vi "Exporting VIs.vi"() -> ()   [LabVIEW 2019]
doc: "This example connects to a server VI that is exporting other VIs through VI Server. It shows how you might browse from one or more applications that may be exporting data from one or more data stations. \n\nThe example shows how to get references to exported VIs and call them with the Call By Reference function."
panel:
  in  "VIs to Export":string="VIs to Export"
  in  "Stop":bool
  out "Data":dbl[](graph)
  in  "Exported VI":i32(listbox)
  # "Overview: Illustrates how to configure and execute Exported VIs in VI Server.\nInstructions:\n1. Ensure Tools > Options > VI Server > Protocols > TCP/IP is enabled, and Port is set to '3363'.\n2. Run the VI. The server VI will open.\n3. Change the Exported VI option below to see the output of different VIs exported by the server displayed in the Data graph.\n4. Click Stop to stop this VI.\n5. Click Stop Server in the server VI to stop the server."
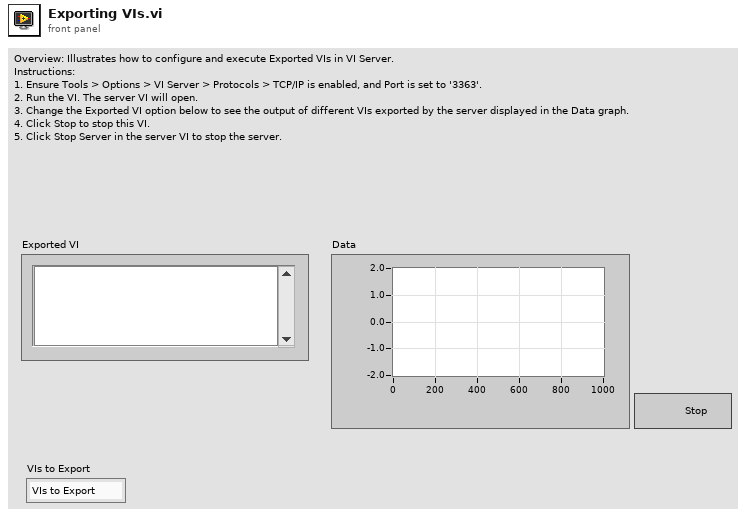
[diagram p1: front panel]
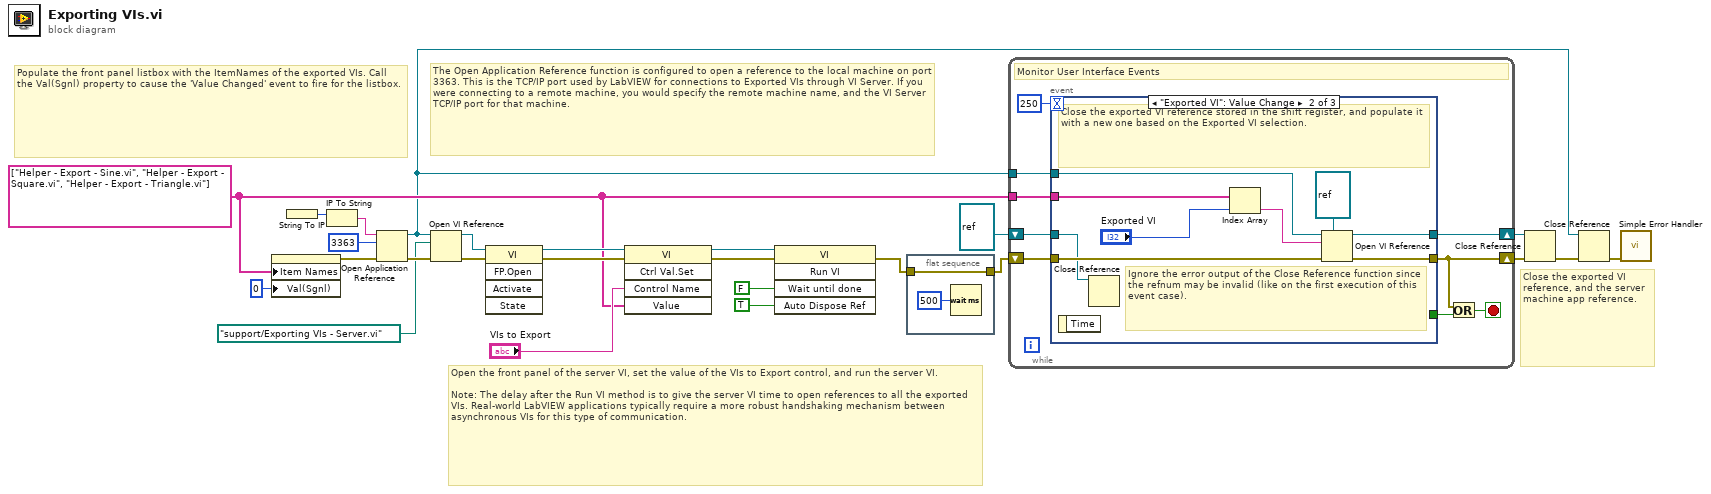
[diagram p0: block diagram]
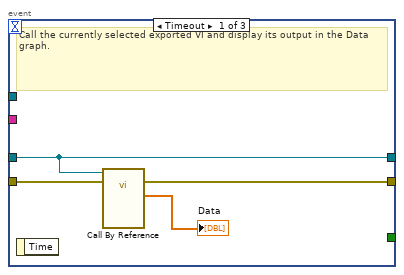
[diagram p2: hidden frame]
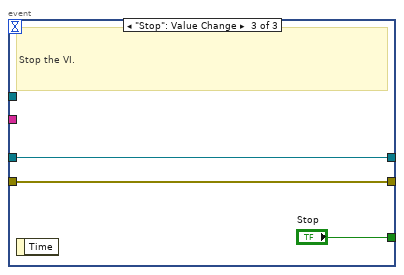
[diagram p3: hidden frame]
diagram:
  w5 = string[] ["Helper - Export - Sine.vi", "Helper - Export - Square.vi", "Helper - Export - Triangle.vi"] ("Exported VI list")
  # "Close the exported VI reference, and the server machine app reference."
  # "The Open Application Reference function is configured to open a reference to the local machine on port 3363. This is the TCP/IP port used by LabVIEW for connections to Exported VIs through VI Server. If you were connecting to a remote machine, you would specify the remote machine name, and the VI Server TCP/IP port for that machine."
  # "Open the front panel of the server VI, set the value of the VIs to Export control, and run the server VI.\n\nNote: The delay after the Run VI method is to give the server VI time to open references to all the exported VIs. Real-world LabVIEW applications typically require a more robust handshaking mechanism between asynchronous VIs for this type of communication."
  # "Populate the front panel listbox with the ItemNames of the exported VIs. Call the Val(Sgnl) property to cause the 'Value Changed' event to fire for the listbox."
  n1 = property on="Exported VI" class="LstBox (strict)"("Item Names"=w5, "Val(Sgnl)"=0 ("Value (Signaling)")) -> (error out=w18:errorcluster)  [unwired: 2 in, 1 out]
  n2 = String To IP() -> (0:w23:u32)  [unwired: 1 in]
  n3 = IP To String(2:w23) -> (0:w17:string)  [unwired: 1 in]
  n4 = Open Application Reference(8:w18, 10:u16 3363 ("VI Server port number"), 11:w17) -> (0:w16:errorcluster, 3:w4:refnum<vi>)  [unwired: 1 out]
  n5 = Open VI Reference(application reference (local)=w4, vi path=path "support/Exporting VIs - Server.vi", error in (no error)=w16) -> (vi reference=w13:refnum<vi>, error out=w14:errorcluster)  [unwired: 3 in]
  n6 = invoke class="VI" method="FP.Open"(reference=w13, error in=w14) -> (reference out=w8:refnum<vi>, error out=w12:errorcluster)  [unwired: 3 in, 3 out]
  n7 = invoke class="VI" method="Ctrl Val.Set"(reference=w8, error in=w12, "Control Name"="VIs to Export", "Value"=w5) -> (reference out=w7:refnum<vi>, error out=w9:errorcluster)  [unwired: 1 in, 3 out]
  n8 = invoke class="VI" method="Run VI"(reference=w7, error in=w9, "Wait until done"=FALSE ("Wait Until Done"), "Auto Dispose Ref"=TRUE ("Auto Dispose Reference")) -> (error out=w2:errorcluster)  [unwired: 1 in, 4 out]
  n9 = flat-sequence {
    tunnel: w2 -> [w27]
    tunnel: [w27] -> w1
    frame #0 {
      n10 = Wait (ms)(milliseconds to wait=u32 500) -> ()  [unwired: 1 out]
    }
  }
  n11 = while {
    shift-left: w1 -> [w34]
    shift-right: [w29] -> w20
    tunnel: w5 -> [w35]
    shift-left: refnum<vi> refnum ("type specifier VI Refnum (for type only)") -> [w32]
    shift-right: [w36] -> w25
    tunnel: w4 -> [w33]
    stop <- w28 stop-if-true
    # "Monitor User Interface Events"
    n12 = event shown="[1] \"Exported VI\": Value Change" {
      selector: _ -> [_ _ _]
      dyn-events: _ -> [_ _ _]
      timeout: 250 -> [_ _ _]
      tunnel: [w39 w49 w51] -> w36
      tunnel: w35 -> [_ w48 _]
      tunnel: w34 -> [w40 w47 w52]
      tunnel: w33 -> [_ w46 _]
      tunnel: [w38 w43 w52] -> w29
      tunnel: w32 -> [w39 w42 w51]
      tunnel: [_ _ "Stop"] -> w30
      event Timeout {
        # "Call the currently selected exported VI and display its output in the Data graph."
        n13 = event-data() -> ()  [unwired: 1 in, 1 out]
        n14 = call-by-ref "?"(reference=w39, error in=w40) -> (error out=w38:errorcluster, "Sine with Noise"=→"Data":dbl[])  [unwired: 11 in, 1 out]
      }
      event "Exported VI": Value Change {
        # "Ignore the error output of the Close Reference function since the refnum may be invalid (like on the first execution of this event case)."
        # "Close the exported VI reference stored in the shift register, and populate it with a new one based on the Exported VI selection."
        n15 = event-data() -> ()  [unwired: 1 in, 1 out]
        n16 = Close Reference(reference=w42) -> ()  [unwired: 1 in, 1 out]
        n17 = Index Array(array=w48, index="Exported VI") -> (element=w44:string)
        n18 = Open VI Reference(type specifier VI Refnum (for type only)=refnum<vi> refnum, application reference (local)=w46, vi path=w44, error in (no error)=w47) -> (vi reference=w49:refnum<vi>, error out=w43:errorcluster)  [unwired: 2 in]
      }
      event "Stop": Value Change {
        # "Stop the VI."
        n19 = event-data() -> ()  [unwired: 1 in, 1 out]
      }
    }
    n20 = Or(x=w29, y=w30) -> (x .or. y?=w28:bool)
  }
  n21 = Close Reference(reference=w25, error in (no error)=w20) -> (error out=w22:errorcluster)
  n22 = Close Reference(reference=w4, error in (no error)=w22) -> (error out=w21:errorcluster)
  n23 = call <vilib>:"Simple Error Handler.vi"("error in (no error)"=w21) -> ()  [unwired: 4 in, 5 out]
